vi "Test Addition.vi"(8 "error in (no error)":errorcluster) -> (0 "error out":errorcluster)   [LabVIEW 2009]
uses:
  classes/Test/Test.lvclass
  classes/Assert/Assert.lvclass
panel:
  # "See block diagram"
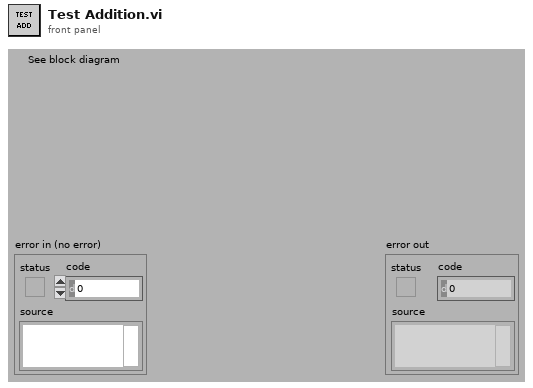
[diagram p1: front panel]
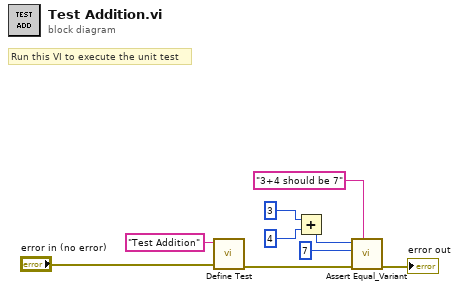
[diagram p0: block diagram]
diagram:
  # "Run this VI to execute the unit test"
  n1 = call "Define Test.vi"("error in (no error)"="error in (no error)", "Label (VI Title)"="Test Addition") -> ("error out"=w4:errorcluster)  [unwired: 9 in]
  n2 = Add(x=3, y=4) -> (x+y=w6:i32)
  n3 = call "Assert Equal_Variant.vi"("Label"="3+4 should be 7", "error in (no error)"=w4, "Y"=7, "X"=w6) -> ("error out"=→"error out":errorcluster)  [unwired: 7 in]
